vi "lidarGetValue.vi"() -> (3 "Lidar_Distance":dbl)   [LabVIEW 2014]
uses:
  Lidar Distance Global.vi
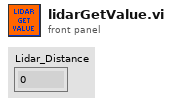
[diagram p1: front panel]
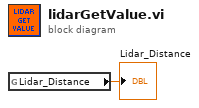
[diagram p0: block diagram]
diagram:
  n1 = global read "Lidar Distance Global.vi" "Lidar_Distance"() -> (→"Lidar_Distance":dbl)
